vi "awg_raw_tcp_control.vi"() -> ()   [LabVIEW 2024]
panel:
  in  "count 2":u16 format="%x"
  in  "commit 2":u32 format="%x"
  in  "gain 2":u32 format="%x"
  in  "index 2":u32=268435460 format="%x"
  in  "count":u16 format="%x"
  in  "commit":u32 format="%x"
  in  "gain":u32 format="%x"
  in  "index":u32=268435460 format="%x"
  out "error out":errorcluster
  # "Frame = [COUNT (2 bytes, big-endian)] + [WORDS]\n\nCOUNT : U16, number of 32-bit words in this frame\n        Example: 0x0003 △ 3 words\n\nWORDS : COUNT ⊙ U32 (big-endian, MSB first)\n        Each word = 32 bits\n        [31:28] = CMD\n        [27]    = Channel (0=A, 1=B)\n        [26:24] = Tone Index (0..7)\n        [23:20] = Reserved\n        [19:0]  = Data (Index/Gain value)\n\nCMD (hex):\n  0x1  △ Set Index\n  0x2  △ Set Gain\n  0xF  △ Commit (apply all previous settings)\n\nIndex value: 0 .. 899        (tone LUT index)\nGain value : 0x00000 .. 0x1FFFF (20-bit Q1.17, full-scale = 0x1FFFF)\n\nExample frame (3 words):\n  COUNT = 0x0003\n  WORD0 = 0x10000001   (Set Index: ch=0, tone=0, index=1)\n  WORD1 = 0x2001FFFF   (Set Gain:  ch=0, tone=0, gain=0x1FFFF)\n  WORD2 = 0xF0000000   (Commit: apply settings)"
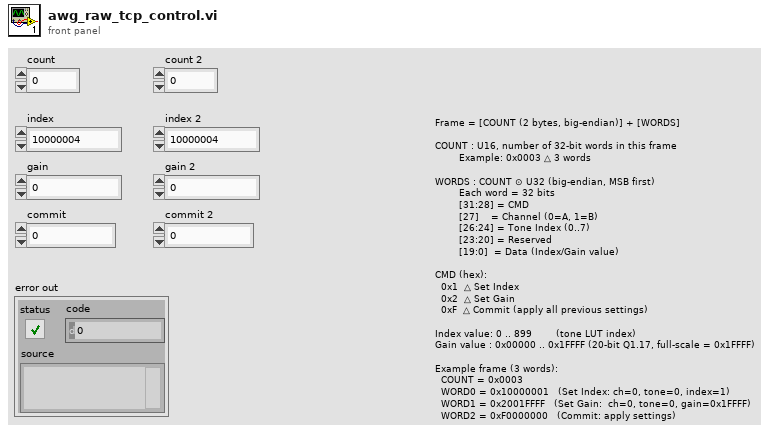
[diagram p1: front panel]
types:
  T1 = enum16{"big-endian, network order", "native, host order", "little-endian"}
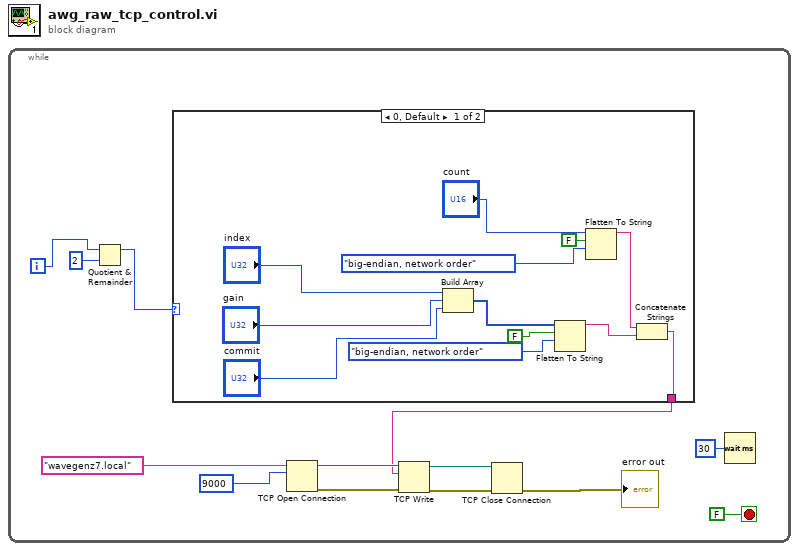
[diagram p0: block diagram]
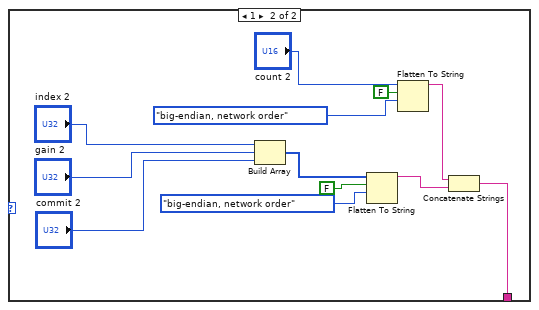
[diagram p2: hidden frame]
diagram:
  n1 = while {
    i -> [w4]
    stop <- FALSE stop-if-true
    n2 = Quotient & Remainder(x=w4, y=i8 2) -> (x-y*floor(x/y)=w3:i32)  [unwired: 1 out]
    n3 = case shown="0, Default" w3 {
      tunnel: [w17 w26] -> w2
      frame 0, Default {
        n4 = Build Array("index", "gain", "commit") -> (w22:u32[])
        n5 = Flatten To String(anything=w22, prepend array or string size? (T)=FALSE, byte order (0:big-endian, network order)=T1."big-endian, network order") -> (data string=w24:string)  [unwired: 1 in, 2 out]
        n6 = Flatten To String(anything="count", prepend array or string size? (T)=FALSE, byte order (0:big-endian, network order)=T1."big-endian, network order") -> (data string=w23:string)  [unwired: 1 in, 2 out]
        n7 = Concatenate Strings(w23, w24) -> (w17:string)
      }
      frame 1 {
        n8 = Build Array("index 2", "gain 2", "commit 2") -> (w31:u32[])
        n9 = Flatten To String(anything=w31, prepend array or string size? (T)=FALSE, byte order (0:big-endian, network order)=T1."big-endian, network order") -> (data string=w33:string)  [unwired: 1 in, 2 out]
        n10 = Flatten To String(anything="count 2", prepend array or string size? (T)=FALSE, byte order (0:big-endian, network order)=T1."big-endian, network order") -> (data string=w32:string)  [unwired: 1 in, 2 out]
        n11 = Concatenate Strings(w32, w33) -> (w26:string)
      }
    }
    n12 = TCP Open Connection(address="wavegenz7.local", remote port or service name=u16 9000) -> (connection ID=w9:refnum<k5>, error out=w10:errorcluster)  [unwired: 3 in]
    n13 = TCP Write(connection ID=w9, data in=w2, error in (no error)=w10) -> (connection ID out=w11:refnum<k5>, error out=w12:errorcluster)  [unwired: 1 in, 1 out]
    n14 = TCP Close Connection(connection ID=w11, error in (no error)=w12) -> (error out=→"error out":errorcluster)  [unwired: 1 in, 1 out]
    n15 = Wait (ms)(milliseconds to wait=u32 30) -> ()  [unwired: 1 out]
  }
